vi "HAL camera stop - SubVI.vi"   [LabVIEW 2014]
uses:
  ATMCD32D.DLL
  camera globals - SubVI.vi
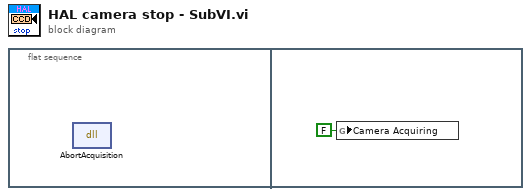
[diagram p0: block diagram]
diagram:
  n1 = flat-sequence {
    frame #0 {
      n2 = dll-call lib="ATMCD32D.DLL" fn="AbortAcquisition" label="Call Library Function\nAbort"() -> ()  [unwired: 3 in, 3 out]
    }
    frame #1 {
      n3 = global write "camera globals - SubVI.vi" "Camera Acquiring"(FALSE ("Andor Aquiring")) -> ()
    }
  }
